vi "svfa_Tone Estimation Subroutine G(f) (first derivative) (complex).vi"(1 "N (window length)":i32=512, 2 "window":T1(ring), 3 "frequency":dbl format="%.5f", 4 "three fingers":cluster{"f0":dbl, "df":dbl, "spectrum":cdb[]}={"f0"=0.0, "df"=1.0, "spectrum"=[]} {"spectrum" format="%.2f"; "df" format="%.2f"; "f0" format="%.2f"}) -> (0 "G'(f)":dbl format="%.2f")   [LabVIEW 2017]
uses:
  <vilib>/addons/_NISVFA/_Spectrum Processing/subVIs/svfa_Tone Estimation Subroutine G(f) (complex).vi
  <vilib>/addons/_NISVFA/_Spectrum Processing/subVIs/svfa_Window Frequency Response.vi
  <vilib>/addons/_NISVFA/_Spectrum Processing/subVIs/svfa_Window Frequency Response (double array).vi
  <vilib>/Analysis/baseanly.llb/Dot Product.vi
  <vilib>/Analysis/baseanly.llb/Complex Dot Product.vi
  <vilib>/addons/_NISVFA/_Spectrum Processing/subVIs/svfa_Rect Window Frequency Response.vi
  <vilib>/addons/_NISVFA/_Spectrum Processing/subVIs/svfa_Cosine Window Coefficients.vi
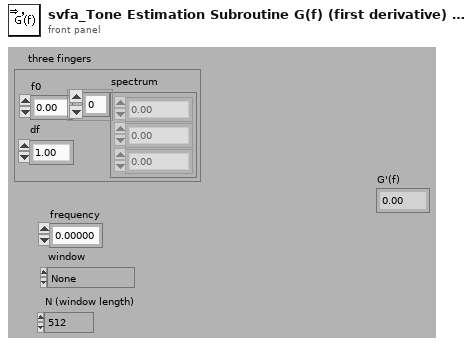
[diagram p1: front panel]
types:
  T1 = enum16{"None ", "Hanning", "Hamming", "Blackman-Harris", "Exact Blackman", "Blackman", "Flat Top", "4 Term B-Harris ", "7 Term B-Harris", "Low Sidelobe"}
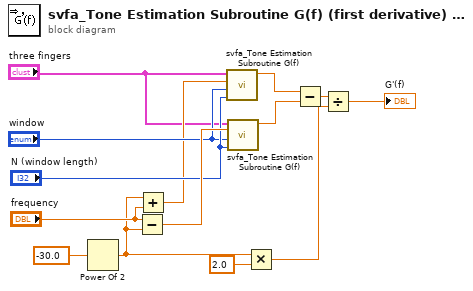
[diagram p0: block diagram]
diagram:
  n1 = Power Of 2(x=-30.0) -> (2^x=w8:dbl)
  n2 = Subtract(x="frequency", y=w8) -> (x-y=w9:dbl)
  n3 = Add(x=w8, y="frequency") -> (x+y=w3:dbl)
  n4 = call-poly <vilib>:"svfa_Tone Estimation Subroutine G(f).vi"("N (window length)"="N (window length)", "window"="window", "frequency"=w3, "three fingers"="three fingers") -> ("G(f)"=w1:dbl)  [unwired: 1 in, 2 out]
  n5 = call-poly <vilib>:"svfa_Tone Estimation Subroutine G(f).vi"("N (window length)"="N (window length)", "window"="window", "frequency"=w9, "three fingers"="three fingers") -> ("G(f)"=w12:dbl)  [unwired: 1 in, 2 out]
  n6 = Multiply(x=w8, y=2.0) -> (x*y=w7:dbl)
  n7 = Subtract(x=w1, y=w12) -> (x-y=w11:dbl)
  n8 = Divide(x=w11, y=w7) -> (x/y=→"G'(f)":dbl)
